vi "XYStage.Home.vi"(8 "error in (no error)":errorcluster, 10 "Wait Timeout, ms (60000)":i32=60000, 11 "XYStage.KIM101 in":refnum<class "XYStage.KIM101.lvclass">) -> (0 "error out":errorcluster, 3 "XYStage.KIM101 out":refnum<class "XYStage.KIM101.lvclass">)   [LabVIEW 2017, in "XYStage.KIM101.lvclass"]
uses:
  XYStage.KIM101.lvclass
  C:/Program Files (x86)/Thorlabs/Kinesis/Thorlabs.MotionControl.KCube.InertialMotorCLI.dll
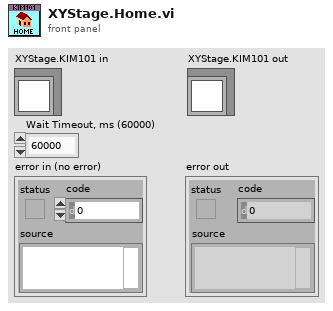
[diagram p1: front panel]
types:
  T1 = typedef "XYStage.KIM101.lvclass/Resource--Cluster.ctl" = cluster{"KCubeInertialMotorControl":refnum<k24>, "Device":refnum<k24>, "X Axis Channel":i32, "Y Axis Channel":i32}
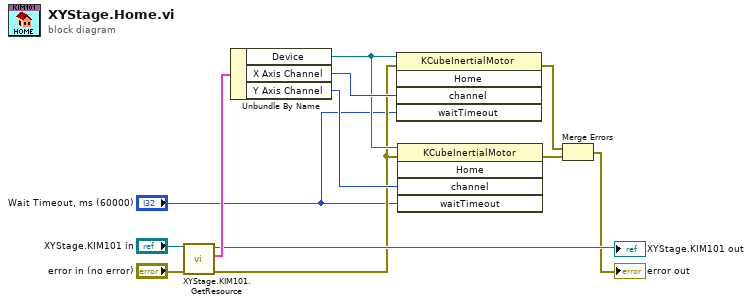
[diagram p0: block diagram]
diagram:
  n1 = call "XYStage.KIM101.GetResource.vi"("error in (no error)"="error in (no error)", "XYStage.KIM101 in"="XYStage.KIM101 in") -> ("error out"=w3:errorcluster, "Resource"=w10:T1, "XYStage.KIM101 out"=→"XYStage.KIM101 out":refnum<class "XYStage.KIM101.lvclass">)  [unwired: 7 in]
  n2 = Unbundle By Name(w10) -> ("Device"=w8:refnum<k24>, "X Axis Channel"=w9:i32, "Y Axis Channel"=w7:i32)
  n3 = invoke class="KCubeInertialMotor" method="Home"(reference=w8, error in=w3, "channel"=w9, "waitTimeout"="Wait Timeout, ms (60000)") -> (error out=w6:errorcluster)  [unwired: 1 in, 4 out]
  n4 = invoke class="KCubeInertialMotor" method="Home"(reference=w8, error in=w3, "channel"=w7, "waitTimeout"="Wait Timeout, ms (60000)") -> (error out=w5:errorcluster)  [unwired: 1 in, 4 out]
  n5 = Merge Errors(w6, w5) -> (→"error out":errorcluster)
